vi "WriteClusterIni.vi"(8 "error in (no error)":errorcluster, 10 "cluster variant":variant=variant(cluster{"test1 (V)":dbl, "Numeric 2":dbl} {"test1 (V)"=424242.0, "Numeric 2"=4442.0}), 11 "configuration file path":path=path "C:/tmp/test.ini") -> (0 "error out":errorcluster, 3 "file path out":path)   [LabVIEW 2018]
uses:
  <vilib>/Utility/config.llb/Write Key (Double).vi
  <vilib>/Utility/config.llb/NI_LVConfig.lvlib
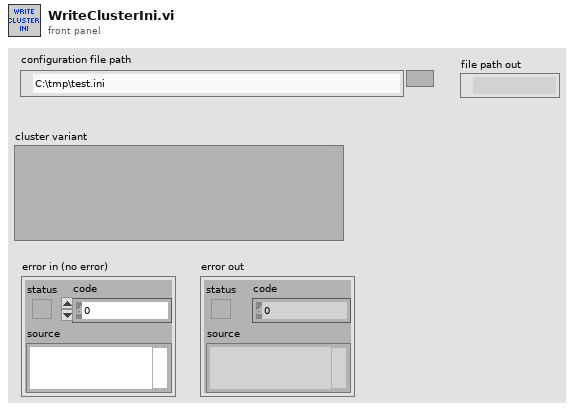
[diagram p1: front panel]
types:
  T1 = typedef "NI_LVConfig.lvlib/Config Data RefNum.ctl" = refnum<k1>
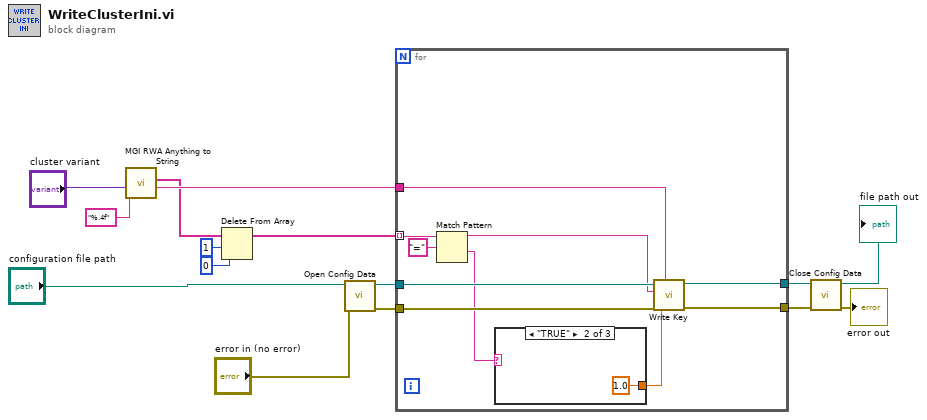
[diagram p0: block diagram]
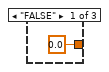
[diagram p2: hidden frame]
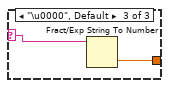
[diagram p3: hidden frame]
diagram:
  n1 = call "MGI RWA Anything to String.vi"("Anything"="cluster variant", "Format String (%#_13g)"="%.4f") -> ("Section"=w12:string, "Strings[]"=w4:string[])  [unwired: 6 in, 2 out]
  n2 = Delete From Array(array=w4, length=1, index=0) -> (array with subset deleted=w2:string[])  [unwired: 1 out]
  n3 = call <vilib>:"Open Config Data.vi"("error in (no error)"="error in (no error)", "configuration file path"="configuration file path") -> ("error out"=w9:errorcluster, "refnum"=w14:T1)  [unwired: 7 in, 1 out]
  n4 = for {
    tunnel: w14 -> [w25]
    tunnel: w2 -> [w24] mode=indexing
    tunnel: [w23] -> w13
    tunnel: w12 -> [w22]
    tunnel: w9 -> [w21]
    tunnel: [w20] -> w8
    n5 = Match Pattern(string=w24, regular expression="=") -> (before substring=w18:string, after substring=w16:string)  [unwired: 1 in, 2 out]
    n6 = case shown="\"TRUE\"" w16 {
      selector: w16 -> [_ _ w28]
      tunnel: [0.0 1.0 w29] -> w17
      frame "FALSE" {
      }
      frame "TRUE" {
      }
      frame "\u0000", Default {
        n7 = Fract/Exp String To Number(string=w28) -> (number=w29:dbl)  [unwired: 3 in, 1 out]
      }
    }
    n8 = call-poly <vilib>:"Write Key.vi"("section"=w22, "error in (no error)"=w21, "value"=w17, "key"=w18, "refnum"=w25) -> ("error out"=w20:errorcluster, "refnum out"=w23:T1)  [unwired: 4 in, 1 out]
  }
  n9 = call <vilib>:"Close Config Data.vi"("error in (no error)"=w8, "refnum"=w13) -> ("error out"=→"error out":errorcluster, "file path"=→"file path out":path)  [unwired: 8 in]
